vi "facade.vi"(0 "Data In":T5, 2 "Display State In":T2={"control refs"={"z offset"=refnum, "laser intensity"=refnum, "XY graph"=refnum}, "error"={"status"=FALSE, "code"=0, "source"=""}, "free-run?"=TRUE, "range (um)"=400, "interpolate?"=FALSE, "settings"={"fix points"=[], "compensation parameters"={"A"=0.0, "lambda"=0.0, "C"=0.0}}}, 3 "Container State":T6) -> (6 "Data Out":T5, 7 "Display State Out":T2={"control refs"={"z offset"=refnum, "laser intensity"=refnum, "XY graph"=refnum}, "error"={"status"=FALSE, "code"=0, "source"=""}, "free-run?"=TRUE, "range (um)"=400, "interpolate?"=FALSE, "settings"={"fix points"=[], "compensation parameters"={"A"=0.0, "lambda"=0.0, "C"=0.0}}}, 8 "Action":T1)   [LabVIEW 2010, in "XIntensityCompensation.xctl"]
uses:
  XIntensityCompensation.xctl
  data.ctl
  <vilib>/_xctls/Container State.ctl
  state.ctl
  control_refs.ctl
  settings_cluster.ctl
  <vilib>/_xctls/Action.ctl
  <vilib>/_xctls/XControlSupport.lvlib
panel:
  in  "loadButton":bool
  in  "saveButton":bool
  in  "C":dbl
  in  "l":dbl[unit]
  in  "A":dbl
  in  "laser intensity (%)":dbl(slide)=14.5 caption="intensity (%)" min=0.001 max=100.0 step=0.1 scale=0.0..100.0 scale format="%.0p"
  in  "depth (z)":dbl[unit](slide) min=0.0 step=1e-07
  in  "addFixPointButton":bool
  in  "clearIntensityPointsButton":bool
  out "depth/intensity set-points":cluster{dbl[unit][], dbl[]}[](graph)
  # "I = A * exp(depth / l) + C"
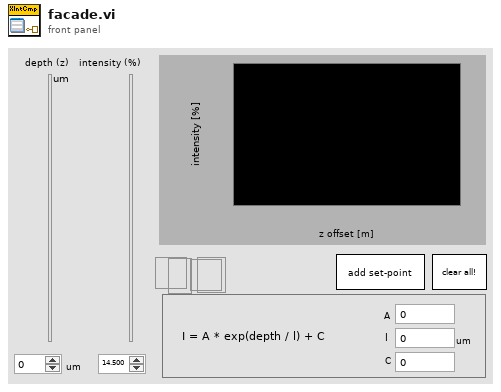
[diagram p1: front panel]
types:
  T1 = typedef "XControlSupport.lvlib/Action.ctl" = cluster{"Data Changed?":bool, "State Changed?":bool, "Action Name":string}
  T2 = typedef "XIntensityCompensation.xctl/state.ctl" = cluster{"control refs":T3, "error":errorcluster, "free-run?":bool, "range (um)":i32, "interpolate?":bool, "settings":T4}
  T3 = typedef "XIntensityCompensation.xctl/control_refs.ctl" = cluster{"z offset":refnum<vi>, "laser intensity":refnum<vi>, "XY graph":refnum<vi>}
  T4 = typedef "XIntensityCompensation.xctl/settings_cluster.ctl" = cluster{"fix points":cluster{"depth":dbl[unit], "intensity":dbl}[], "compensation parameters":T5}
  T5 = typedef "XIntensityCompensation.xctl/data.ctl" = cluster{"A":dbl, "lambda":dbl[unit], "C":dbl}
  T6 = typedef "XControlSupport.lvlib/Container State.ctl" = cluster{"Indicator?":bool, "Run Mode?":bool, " Refnum":refnum<vi>}
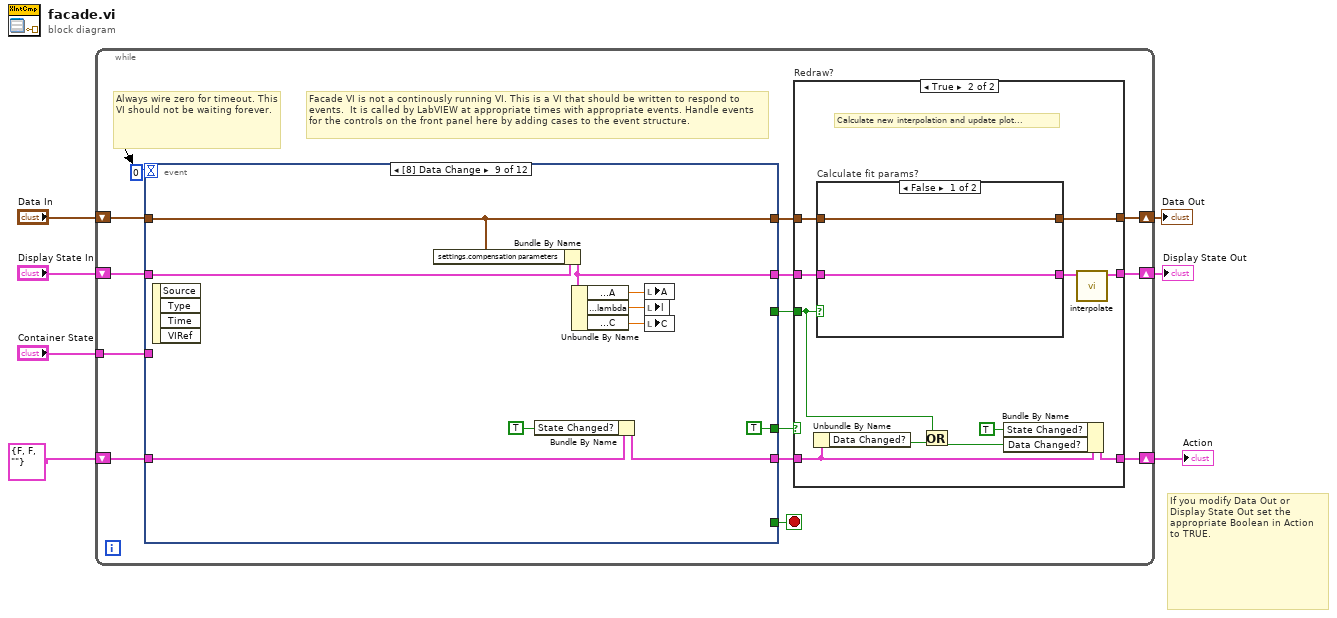
[diagram p0: block diagram]
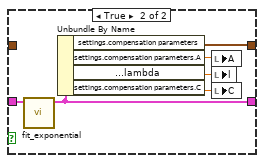
[diagram p3: hidden frame]
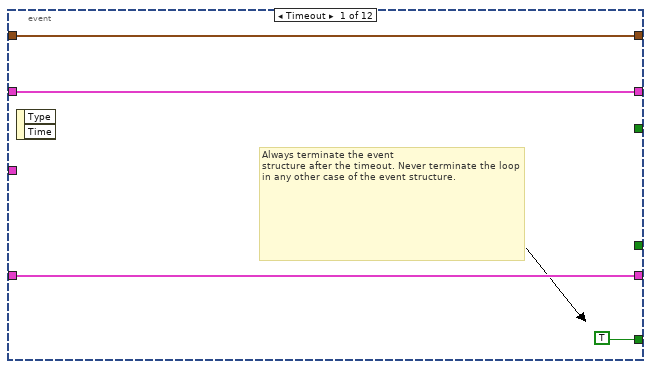
[diagram p4: hidden frame]
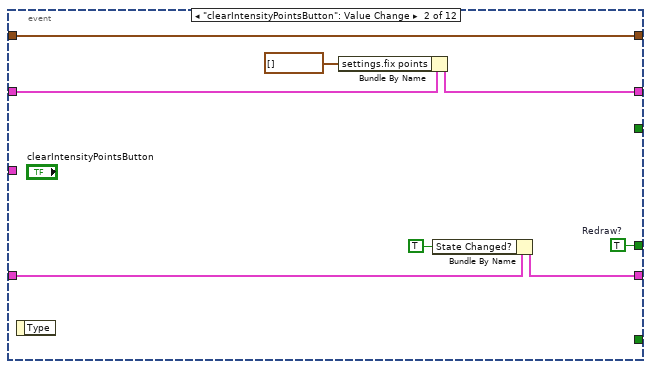
[diagram p5: hidden frame]
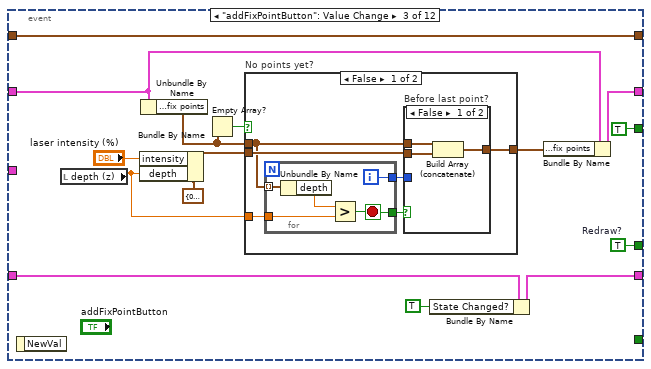
[diagram p6: hidden frame]
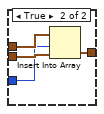
[diagram p7: hidden frame]
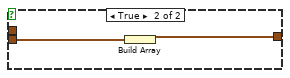
[diagram p8: hidden frame]
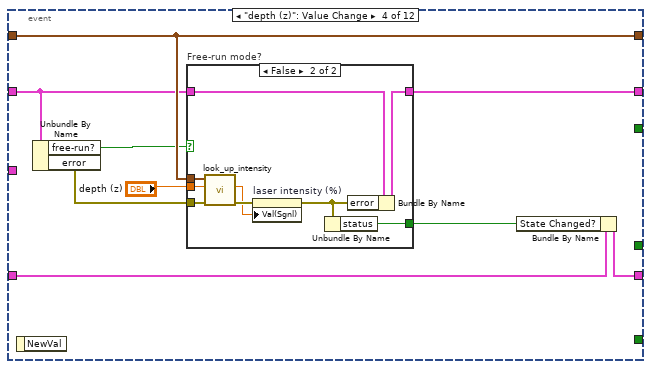
[diagram p9: hidden frame]
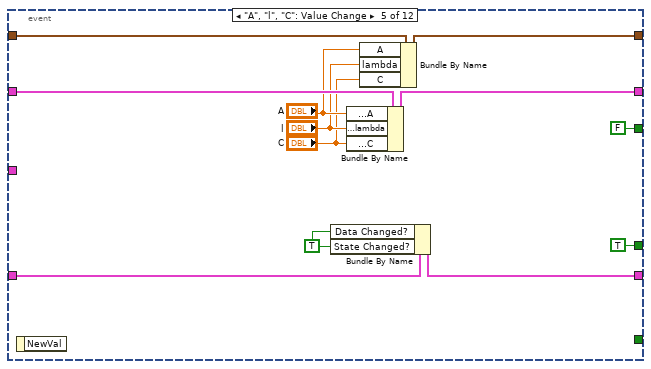
[diagram p11: hidden frame]
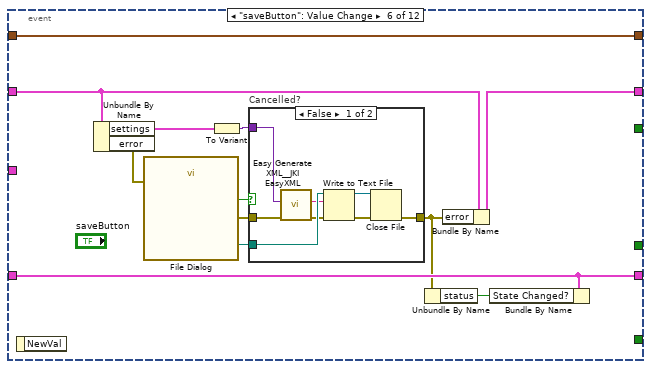
[diagram p12: hidden frame]
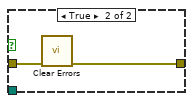
[diagram p13: hidden frame]
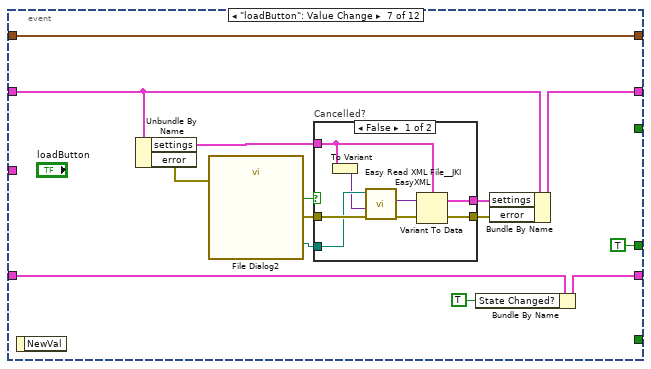
[diagram p14: hidden frame]
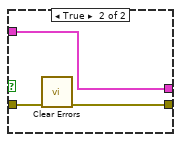
[diagram p15: hidden frame]
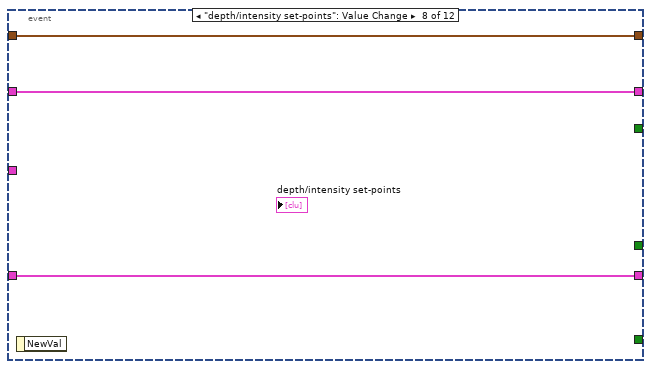
[diagram p16: hidden frame]
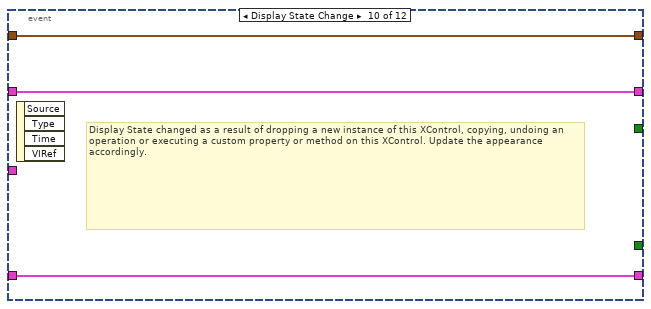
[diagram p17: hidden frame]
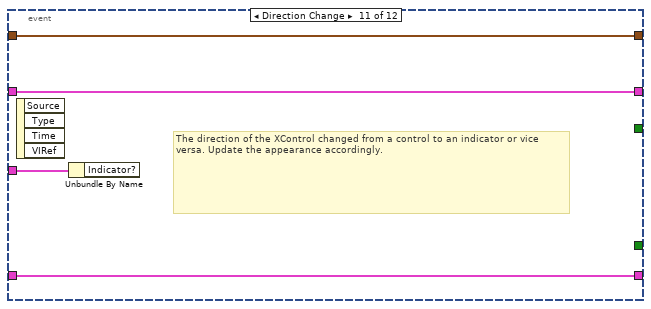
[diagram p18: hidden frame]
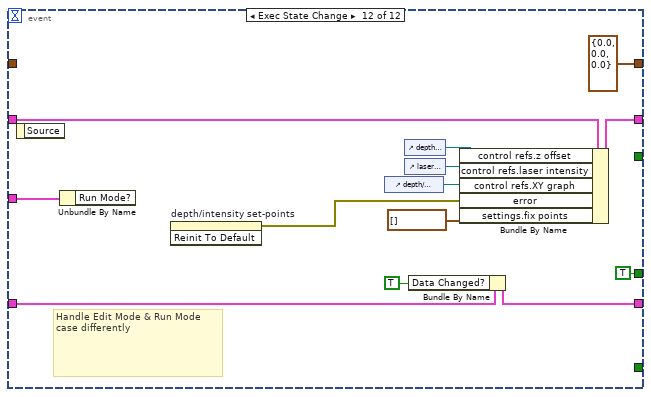
[diagram p19: hidden frame]
diagram:
  # "If you modify Data Out or\nDisplay State Out set the\nappropriate Boolean in Action\nto TRUE."
  n1 = while {
    shift-right: [w15] -> w5
    shift-left: "Display State In" -> [w21]
    tunnel: "Container State" -> [w18]
    shift-right: [w11] -> w1
    shift-left: "Data In" -> [w17]
    shift-right: [w13] -> w3
    shift-left: T1 {"Data Changed?"=FALSE, "State Changed?"=FALSE, "Action Name"=""} ("Action") -> [w16]
    stop <- w20 stop-if-true
    # "Facade VI is not a continously running VI. This is a VI that should be written to respond to events.  It is called by LabVIEW at appropriate times with appropriate events. Handle events for the controls on the front panel here by adding cases to the event structure."
    # "Always wire zero for timeout. This\nVI should not be waiting forever."
    n2 = event shown="[8] Data Change" {
      selector: _ -> [_ _ _ _ _ _ _ _ _ _ _ _]
      dyn-events: _ -> [_ _ _ _ _ _ _ _ _ _ _ _]
      timeout: 0 -> [_ _ _ _ _ _ _ _ _ _ _ _]
      tunnel: w21 -> [w45 w53 w63 w96 w121 w126 w148 w171 w180 w184 w187 w200]
      tunnel: [w45 w52 w66 w92 w120 w131 w152 w171 w176 w184 w187 w199] -> w9
      tunnel: [TRUE _ _ _ _ _ _ _ _ _ _ _] -> w20
      tunnel: w18 -> [_ _ _ _ _ _ _ _ _ _ w188 w201]
      tunnel: w17 -> [w44 w54 w67 w97 w111 w133 w157 w170 w181 w183 w186 _]
      tunnel: [w44 w54 w67 w97 w110 w133 w157 w170 w181 w183 w186 T5 {"A"=0.0, "lambda"=0.0, "C"=0.0} ("fix points")] -> w12
      tunnel: [w46 w49 w56 w93 w118 w124 w144 w169 w172 w182 w185 w189] -> w10
      tunnel: w16 -> [w46 w50 w57 w94 w119 w124 w145 w169 w173 w182 w185 w190]
      tunnel: [_ w48 w64 _ TRUE ("Data Changed?") _ TRUE ("Data Changed?") _ TRUE ("Data Changed?") _ _ TRUE ("Data Changed?")] -> w14
      tunnel: [_ _ TRUE _ FALSE _ _ _ _ _ _ _] -> w8
      event Timeout {
        # "Always terminate the event\nstructure after the timeout. Never terminate the loop in any other case of the event structure."
        n3 = event-data() -> ()  [unwired: 1 in, 2 out]
      }
      event "clearIntensityPointsButton": Value Change {
        w48 = TRUE  # Redraw?
        n4 = event-data() -> ()  [unwired: 1 in, 1 out]
        n5 = Bundle By Name(cluster=w53, "settings.fix points"=cluster{"depth":dbl[unit], "intensity":dbl}[] [] ("fix points")) -> (w52:T2)
        n6 = Bundle By Name(cluster=w50, "State Changed?"=TRUE) -> (w49:T1)
      }
      event "addFixPointButton": Value Change {
        w64 = TRUE  # Redraw?
        n7 = event-data() -> ()  [unwired: 1 in, 1 out]
        n8 = local read "depth (z)"() -> (w60:dbl[unit])
        n9 = Bundle By Name(cluster=cluster{"depth":dbl[unit], "intensity":dbl} {"depth"=0.0, "intensity"=0.0} ("intensity/depth combination"), "intensity"="laser intensity (%)", "depth"=w60) -> (w69:cluster{"depth":dbl[unit], "intensity":dbl})
        n10 = Unbundle By Name(w63) -> ("settings.fix points"=w62:cluster{"depth":dbl[unit], "intensity":dbl}[])
        n11 = Empty Array?(array=w62) -> (empty?=w61:bool)
        n12 = case "No points yet?" shown="False" w61 {
          tunnel: w69 -> [w76 w90]
          tunnel: w60 -> [w75 _]
          tunnel: w62 -> [w74 _]
          tunnel: [w73 w89] -> w65
          frame False {
            n13 = for {
              tunnel: w74 -> [w88] mode=indexing
              tunnel: w75 -> [w85]
              tunnel: [w87] -> w71
              tunnel: [w86] -> w72
              i -> [w87]
              stop <- w86 stop-if-true
              n14 = Unbundle By Name(w88) -> ("depth"=w84:dbl[unit])
              n15 = Greater?(x=w84, y=w85) -> (0:w86:bool)
            }
            n16 = case "Before last point?" shown="False" w72 {
              tunnel: w76 -> [w77 w83]
              tunnel: [w78 w82] -> w73
              tunnel: w74 -> [w79 w81]
              tunnel: w71 -> [_ w80]
              frame False {
                n17 = Build Array (concatenate)(w79, w77) -> (w78:cluster{"depth":dbl[unit], "intensity":dbl}[])
              }
              frame True {
                n18 = Insert Into Array(array=w81, index=w80, new element=w83) -> (w82:cluster{"depth":dbl[unit], "intensity":dbl}[])
              }
            }
          }
          frame True {
            n19 = Build Array(w90) -> (w89:cluster{"depth":dbl[unit], "intensity":dbl}[])
          }
        }
        n20 = Bundle By Name(cluster=w57, "State Changed?"=TRUE) -> (w56:T1)
        n21 = Bundle By Name(cluster=w63, "settings.fix points"=w65) -> (w66:T2)
      }
      event "depth (z)": Value Change {
        n22 = event-data() -> ()  [unwired: 1 in, 1 out]
        n23 = Unbundle By Name(w96) -> ("free-run?"=w95:bool, "error"=w99:errorcluster)
        n24 = case "Free-run mode?" shown="False" w95 {
          tunnel: w99 -> [_ w109]
          tunnel: "depth (z)" -> [_ w108]
          tunnel: w97 -> [_ w107]
          tunnel: w96 -> [w100 w104]
          tunnel: [w100 w103] -> w92
          tunnel: [_ w101] -> w91
          frame True {
          }
          frame False {
            n25 = call "look_up_intensity.vi"("error in (no error)"=w109, "z offset"=w108, "compensation parameters"=w107) -> ("error out"=w106:errorcluster, "intensity"=w105:dbl)  [unwired: 7 in]
            n26 = property on="laser intensity (%)" class="Slide (strict)"(error in=w106, "Val(Sgnl)"=w105) -> (error out=w102:errorcluster)  [unwired: 1 in, 1 out]
            n27 = Unbundle By Name(w102) -> ("status"=w101:bool)
            n28 = Bundle By Name(cluster=w104, "error"=w102) -> (w103:T2)
          }
        }
        n29 = Bundle By Name(cluster=w94, "State Changed?"=w91) -> (w93:T1)
      }
      event "A", "l", "C": Value Change {
        w115 = TRUE ("State Changed?")
        n30 = event-data() -> ()  [unwired: 1 in, 1 out]
        n31 = Bundle By Name(cluster=w119, "Data Changed?"=w115, "State Changed?"=w115) -> (w118:T1)
        n32 = Bundle By Name(cluster=w121, "settings.compensation parameters.A"="A", "settings.compensation parameters.lambda"="l", "settings.compensation parameters.C"="C") -> (w120:T2)
        n33 = Bundle By Name(cluster=w111, "A"="A", "lambda"="l", "C"="C") -> (w110:T5)
      }
      event "saveButton": Value Change {
        n34 = event-data() -> ()  [unwired: 1 in, 1 out]
        n35 = Unbundle By Name(w126) -> ("settings"=w132:T4, "error"=w130:errorcluster)
        n36 = call "File Dialog"("error in"=w130) -> ("selected path"=w128:path, "cancelled"=w125:bool, "error out"=w129:errorcluster)  [unwired: 11 in, 1 out]
        n37 = To Variant(anything=w132) -> (Variant=w127:variant)
        n38 = case "Cancelled?" shown="False" w125 {
          tunnel: [w134 w142] -> w123
          tunnel: w129 -> [w140 w143]
          tunnel: w128 -> [w139 _]
          tunnel: w127 -> [w141 _]
          frame False {
            n39 = call <vilib>:"Easy Generate XML__JKI EasyXML.vi"("error in (no error)"=w140, "LabVIEW Data"=w141) -> ("error out"=w138:errorcluster, "XML String"=w137:string)  [unwired: 1 in, 7 out]
            n40 = Write to Text File(file (use dialog)=w139, text=w137, error in=w138) -> (refnum out=w136:refnum<file>, error out=w135:errorcluster)  [unwired: 2 out]
            n41 = Close File(refnum=w136, error in=w135) -> (error out=w134:errorcluster)  [unwired: 1 out]
          }
          frame True {
            n42 = call <vilib>:"Clear Errors.vi"("error in (no error)"=w143) -> ("error out"=w142:errorcluster)  [unwired: 6 in]
          }
        }
        n43 = Unbundle By Name(w123) -> ("status"=w122:bool)
        n44 = Bundle By Name(cluster=w126, "error"=w123) -> (w131:T2)
        n45 = Bundle By Name(cluster=w124, "State Changed?"=w122) -> ()  [unwired: 1 out]
      }
      event "loadButton": Value Change {
        n46 = event-data() -> ()  [unwired: 1 in, 1 out]
        n47 = Unbundle By Name(w148) -> ("settings"=w150:T4, "error"=w156:errorcluster)
        n48 = call "File Dialog2"("error in"=w156) -> ("selected path"=w154:path, "cancelled"=w153:bool, "error out"=w155:errorcluster)  [unwired: 11 in, 1 out]
        n49 = case "Cancelled?" shown="False" w153 {
          tunnel: [w162 w167] -> w151
          tunnel: w155 -> [w165 w168]
          tunnel: w154 -> [w164 _]
          tunnel: w150 -> [w158 w166]
          tunnel: [w159 w166] -> w149
          frame False {
            n50 = To Variant(anything=w158) -> (Variant=w160:variant)
            n51 = call <vilib>:"Easy Read XML File__JKI EasyXML.vi"("error in (no error)"=w165, "LabVIEW Data (Type)"=w160, "XML File Path"=w164) -> ("error out"=w163:errorcluster, "LabVIEW Data"=w161:variant)  [unwired: 6 in, 1 out]
            n52 = Variant To Data(error in=w163, Variant=w161, type=w158) -> (error out=w162:errorcluster, data=w159:T4)
          }
          frame True {
            n53 = call <vilib>:"Clear Errors.vi"("error in (no error)"=w168) -> ("error out"=w167:errorcluster)  [unwired: 6 in]
          }
        }
        n54 = Bundle By Name(cluster=w145, "State Changed?"=TRUE) -> (w144:T1)
        n55 = Bundle By Name(cluster=w148, "settings"=w149, "error"=w151) -> (w152:T2)
      }
      event "depth/intensity set-points": Value Change {
        n56 = event-data() -> ()  [unwired: 1 in, 1 out]
      }
      event Data Change {
        n57 = event-data() -> ()  [unwired: 1 in, 4 out]
        n58 = Bundle By Name(cluster=w180, "settings.compensation parameters"=w181) -> (w176:T2)
        n59 = Bundle By Name(cluster=w173, "State Changed?"=TRUE ("Data Changed?")) -> (w172:T1)
        n60 = Unbundle By Name(w176) -> ("settings.compensation parameters.A"=w177:dbl, "settings.compensation parameters.lambda"=w179:dbl[unit], "settings.compensation parameters.C"=w178:dbl)
        n61 = local write "A"(w177) -> ()
        n62 = local write "l"(w179) -> ()
        n63 = local write "C"(w178) -> ()
      }
      event Display State Change {
        # "Display State changed as a result of dropping a new instance of this XControl, copying, undoing an operation or executing a custom property or method on this XControl. Update the appearance accordingly."
        n64 = event-data() -> ()  [unwired: 1 in, 4 out]
      }
      event Direction Change {
        # "The direction of the XControl changed from a control to an indicator or vice versa. Update the appearance accordingly."
        n65 = event-data() -> ()  [unwired: 1 in, 4 out]
        n66 = Unbundle By Name(w188) -> ()  [unwired: 1 out]
      }
      event Exec State Change {
        # "Handle Edit Mode & Run Mode\ncase differently"
        n67 = event-data() -> ()  [unwired: 1 in, 1 out]
        n68 = Unbundle By Name(w201) -> ()  [unwired: 1 out]
        n69 = invoke on="depth/intensity set-points" class="XYGraph (strict)" method="Reinit To Default"() -> (error out=w192:errorcluster)  [unwired: 3 in, 2 out]
        n70 = control-ref of="depth/intensity set-points"() -> (w194:refnum<vi>)
        n71 = control-ref of="depth (z)"() -> (w198:refnum<vi>)
        n72 = control-ref of="laser intensity (%)"() -> (w197:refnum<vi>)
        n73 = Bundle By Name(cluster=w190, "Data Changed?"=TRUE) -> (w189:T1)
        n74 = Bundle By Name(cluster=w200, "control refs.z offset"=w198, "control refs.laser intensity"=w197, "control refs.XY graph"=w194, "error"=w192, "settings.fix points"=cluster{"depth":dbl[unit], "intensity":dbl}[] []) -> (w199:T2)
      }
    }
    n75 = case "Redraw?" shown="True" w14 {
      tunnel: [w24 w30] -> w15
      tunnel: w9 -> [w24 w34]
      tunnel: w10 -> [w22 w28]
      tunnel: [w22 w35] -> w13
      tunnel: w12 -> [w23 w32]
      tunnel: [w23 w31] -> w11
      tunnel: w8 -> [_ w25]
      frame False {
      }
      frame True {
        # "Calculate new interpolation and update plot..."
        n76 = Unbundle By Name(w28) -> ("Data Changed?"=w26:bool)
        n77 = case "Calculate fit params?" shown="False" w25 {
          tunnel: w34 -> [w37 w43]
          tunnel: [w37 w39] -> w33
          tunnel: w32 -> [w36 _]
          tunnel: [w36 w38] -> w31
          frame False {
          }
          frame True {
            n78 = call "fit_exponential.vi"("State in"=w43) -> ("State out"=w39:T2)  [unwired: 10 in]
            n79 = Unbundle By Name(w39) -> ("settings.compensation parameters"=w38:T5, "settings.compensation parameters.A"=w42:dbl, "settings.compensation parameters.lambda"=w40:dbl[unit], "settings.compensation parameters.C"=w41:dbl)
            n80 = local write "A"(w42) -> ()
            n81 = local write "l"(w40) -> ()
            n82 = local write "C"(w41) -> ()
          }
        }
        n83 = Or(x=w25, y=w26) -> (x .or. y?=w27:bool)
        n84 = Bundle By Name(cluster=w28, "State Changed?"=TRUE, "Data Changed?"=w27) -> (w35:T1)
        n85 = call "interpolate.vi"("State in"=w33) -> ("State out"=w30:T2)  [unwired: 10 in]
      }
    }
  }
  "Display State Out" <- w5
  "Data Out" <- w1
  "Action" <- w3
